vi "Open waveform write sessions.vi"(7 "Already opened?":bool, 8 "error in (no error)":errorcluster, 9 "ChannelOuputs In":dbl[](array[numeric]), 10 "Device Outputs FIFO":refnum<k33>, 11 "Multiple Waveforms Write Session (DBL)":refnum<class "Multiple Waveforms Write (DBL).lvclass">) -> (0 "error out":errorcluster, 1 "ChannelOuputs Out":dbl[](array[numeric]), 3 "Multiple Waveforms Write Session (DBL)":refnum<class "Multiple Waveforms Write (DBL).lvclass">, 5 "Opened":bool)   [LabVIEW 2013, in "Waveforms Generation Custom Device.lvlib"]
uses:
  Waveforms Generation Custom Device.lvlib
  <vilib>/NI Veristand/Custom Device Waveform API/Multiple Waveforms Write (DBL)/Multiple Waveforms Write (DBL).lvclass
  <vilib>/NI Veristand/Custom Device Waveform API/Waveform Session.lvclass/Waveform Session.ctl
  <vilib>/NI Veristand/Custom Device Waveform API/Multiple Waveforms Write (DBL)/Multiple Waveforms Write (DBL).lvclass/Multiple Waveforms Write (DBL).ctl
  <vilib>/NI Veristand/Custom Device Waveform API/Internal Comm Classes/WPL Comm/WPL Comm.lvclass/WPL Comm.ctl
  <vilib>/NI Veristand/Custom Device Waveform API/Multiple Waveforms Write (DBL)/NI VeriStand - Start Multiple Waveforms (DBL).vi
  <vilib>/NI Veristand/Custom Device Waveform API/Internal Comm Classes/WPL Comm/WPL_start dbl waveform.vi
  <vilib>/NI Veristand/Custom Device Waveform API/Read Sample offset DVR.vi
  <vilib>/NI Veristand/Custom Device Waveform API/Check Opened.vi
  <vilib>/NI Veristand/Custom Device Waveform API/Internal Comm Classes/WPL Comm/Set t0 on Variant.vi
  <vilib>/NI Veristand/Custom Device Waveform API/Internal Comm Classes/WPL Comm/Send WPL Command.vi
  <vilib>/NI Veristand/Custom Device Waveform API/Internal Comm Classes/WPL Comm/Convert Q Error to Shutdown Error.vi
  <vilib>/Utility/error.llb/Error Cluster From Error Code.vi
  <vilib>/NI Veristand/Custom Device Waveform API/NI_VS Custom Device Waveform API.lvlib
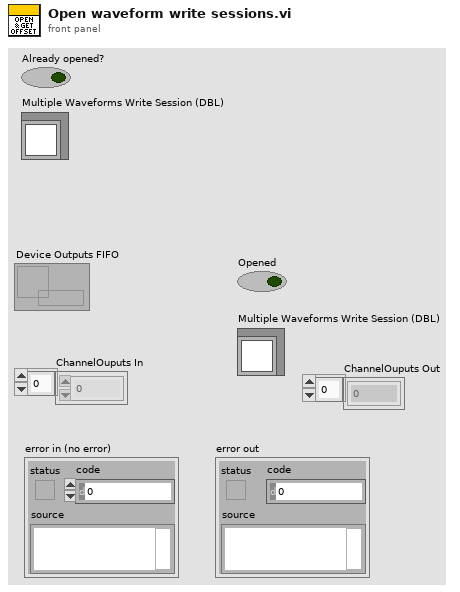
[diagram p1: front panel]
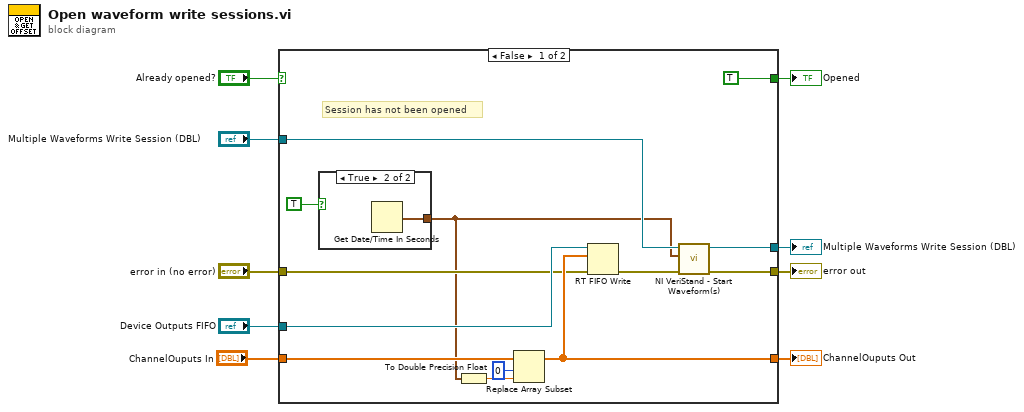
[diagram p0: block diagram]
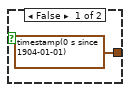
[diagram p2: hidden frame]
diagram:
  n1 = case shown="False" "Already opened?" {
    selector: "Already opened?" -> [_ w27]
    tunnel: "error in (no error)" -> [w13 w28]
    tunnel: [w21 w28] -> w9
    tunnel: [TRUE ("Filter FIFO Errors (T)") w27] -> w7
    tunnel: [w20 w26] -> w5
    tunnel: "Multiple Waveforms Write Session (DBL)" -> [w19 w26]
    tunnel: "Device Outputs FIFO" -> [w17 _]
    tunnel: "ChannelOuputs In" -> [w16 w25]
    tunnel: [w14 w25] -> w1
    frame False {
      # "Session has not been opened"
      n2 = case shown="True" TRUE {
        tunnel: [timestamp(0 s since 1904-01-01) ("seconds since 1Jan1904") w24] -> w10
        frame False {
        }
        frame True {
          n3 = Get Date/Time In Seconds() -> (seconds since 1Jan1904=w24:timestamp)
        }
      }
      n4 = To Double Precision Float(number=w10) -> (double precision float=w11:dbl)
      n5 = Replace Array Subset(array=w16, new element=w11, index=0) -> (w14:dbl[])
      n6 = RT FIFO Write(0:w17, 1:w14, 3:w13) -> (11:w12:errorcluster)  [unwired: 2 in, 3 out]
      n7 = call-poly <vilib>:"NI VeriStand - Start Waveform(s).vi"("error in (no error)"=w12, "t0"=w10, "Multiple Waveforms Write Session (DBL) in"=w19) -> ("error out"=w21:errorcluster, "Multiple Waveforms Write Session (DBL) out"=w20:refnum<class "Multiple Waveforms Write (DBL).lvclass">)  [unwired: 7 in]
    }
    frame True {
      # "Write session was already opened."
    }
  }
  "error out" <- w9
  "Opened" <- w7
  "Multiple Waveforms Write Session (DBL)" <- w5
  "ChannelOuputs Out" <- w1
